vi "MotorPowerShaper.vi"(5 "JoystickValues":dbl[](array[numeric])=[0.0, 0.0, 0.0], 6 "Third Speed":bool, 7 "Shaping Degree":dbl=3.0, 8 "Gain":dbl=50.0, 9 "Position":dbl=-2819.0, 10 "Power":dbl, 11 "Setpoint":dbl=-2900.7999999999997) -> (2 "Power Out":dbl, 3 "Setpoint Out":dbl=-2818.6092010617926)   [LabVIEW 2014]
uses:
  <vilib>/Rock Robotics/WPI/Joystick/WPI_JoystickGetSetRefNum.vi
panel:
  in  "Error Deviation":dbl=400.0
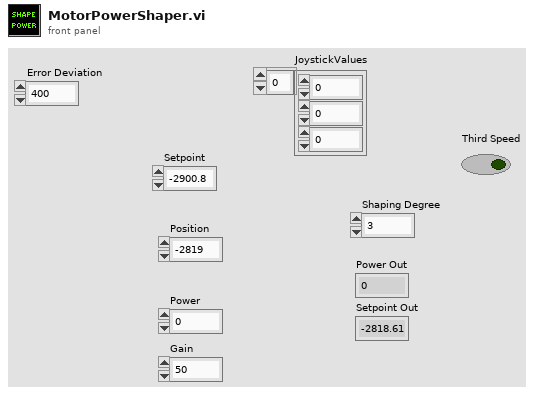
[diagram p1: front panel]
types:
  T1 = typedef "WPI_JoystickDevRef.ctl" = cluster{"Device":T2}
  T2 = typedef "WPI_JoystickDeviceEnum.ctl" = enum16{"USB 0", "USB 1", "USB 2", "USB 3", "USB 4", "USB 5"}
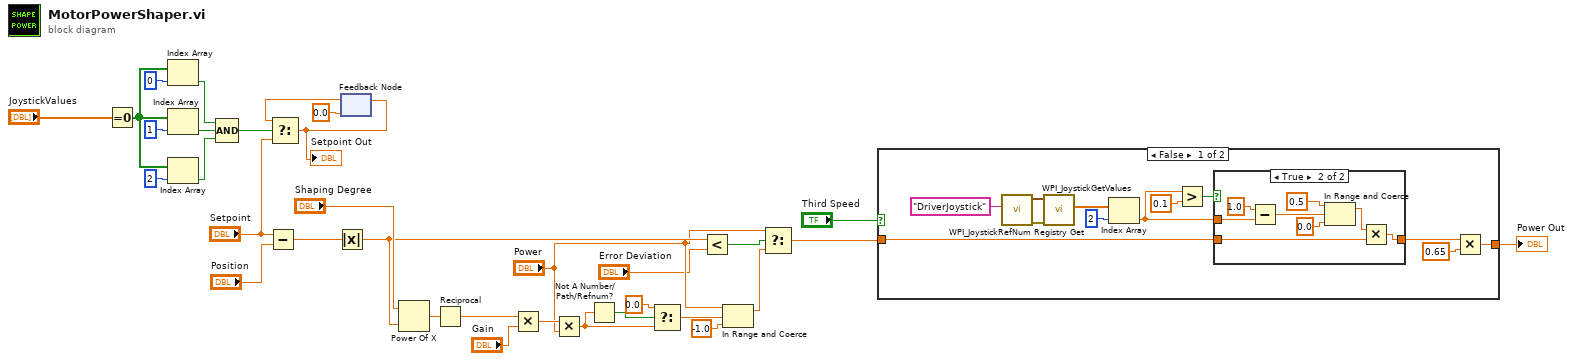
[diagram p0: block diagram]
diagram:
  n1 = Equal To 0?(x="JoystickValues") -> (x = 0?=w14:bool[])
  n2 = Index Array(array=w14, index=0) -> (element=w15:bool)
  n3 = Index Array(array=w14, index=1) -> (element=w11:bool)
  n4 = Index Array(array=w14, index=2) -> (element=w10:bool)
  n5 = Compound Arithmetic op=AND(w15, w11, w10) -> (w9:bool)
  n6 = Subtract(x="Setpoint", y="Position") -> (x-y=w32:dbl)
  n7 = Absolute Value(x=w32) -> (abs(x)=w21:dbl)
  n8 = feedback #1(0.0 ("t")) -> (w8:dbl)
  n9 = Select(t=w8, s=w9, f="Setpoint") -> (s? t:f=w5:dbl)
  "Setpoint Out" <- w5
  n10 = feedback-in #1(w5) -> ()
  n11 = Power Of X(1:w21, 2:"Shaping Degree") -> (0:w31:dbl)
  n12 = Reciprocal(x=w31) -> (1/x=w30:dbl)
  n13 = Multiply(x=w30, y="Gain") -> (x*y=w28:dbl)
  n14 = Multiply(x=w28, y="Power") -> (x*y=w24:dbl)
  n15 = Not A Number/Path/Refnum?(number/path/refnum=w24) -> (NaN/Path/Refnum?=w26:bool)
  n16 = Select(t=0.0, s=w26, f=w24) -> (s? t:f=w22:dbl)
  n17 = Less?(x=w21, y="Error Deviation") -> (x < y?=w20:bool)
  n18 = In Range and Coerce(upper limit="Power", x=w22, lower limit=-1.0) -> (coerced(x)=w18:dbl)  [unwired: 1 out]
  n19 = Select(t="Power", s=w20, f=w18) -> (s? t:f=w1:dbl)
  n20 = case shown="False" "Third Speed" {
    tunnel: w1 -> [w38 w55]
    tunnel: [w36 w55] -> w4
    frame False {
      n21 = call <vilib>:"WPI_JoystickRefNum Registry Get.vi"("refnum name"="DriverJoystick") -> ("error out"=w43:errorcluster, "JoystickDevRef"=w42:T1)  [unwired: 9 in]
      n22 = call <vilib>:"WPI_JoystickGetValues.vi"("error in (no error)"=w43, "JoystickDevRef"=w42) -> ("Axes"=w45:dbl[])  [unwired: 5 in, 4 out]
      n23 = Index Array(array=w45, index=2) -> (element=w34:dbl)
      n24 = Greater?(x=w34, y=0.1) -> (0:w39:bool)
      n25 = case shown="True" w39 {
        tunnel: w38 -> [w46 w49]
        tunnel: [w46 w48] -> w37
        tunnel: w34 -> [_ w47]
        frame False {
        }
        frame True {
          n26 = Subtract(x=1.0 ("upper limit"), y=w47) -> (x-y=w54:dbl)
          n27 = In Range and Coerce(upper limit=0.5, x=w54, lower limit=0.0) -> (coerced(x)=w50:dbl)  [unwired: 1 out]
          n28 = Multiply(x=w50, y=w49) -> (x*y=w48:dbl)
        }
      }
      n29 = Multiply(x=w37, y=0.65) -> (x*y=w36:dbl)
    }
    frame True {
    }
  }
  "Power Out" <- w4
